vi "RP Read Subset VISA.vi"(6 "Bytes per sample":i32, 7 "Samples per trigger increment":i32=2, 8 "Error In":errorcluster, 9 "Post-trigger samples":u64=11534336 format="0x%x (%d)", 10 "Pre-trigger samples":i32=-100000 format="0x%x (%d)", 11 "VISA resource":refnum<visa-resource-name>) -> (0 "Error Out":errorcluster, 1 "Record start pos":u32=1, 2 "Data stream":string, 3 "VISA resource out":refnum<visa-resource-name>)   [LabVIEW 2024]
uses:
  RP Command.ctl
  RP Status Offsets.ctl
  RP Read Status VISA.vi
  RP Write Command VISA.vi
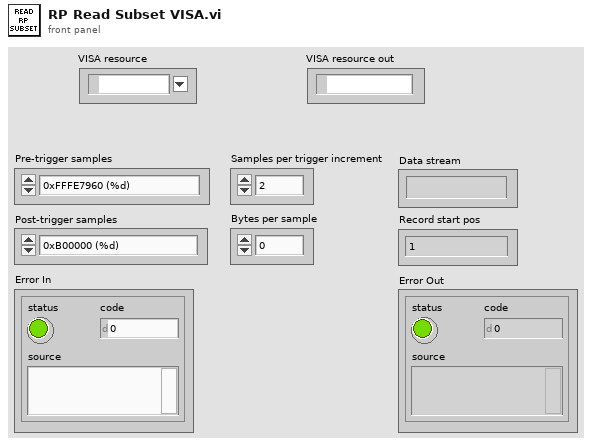
[diagram p1: front panel]
types:
  T1 = typedef "RP Status Offsets.ctl" = u16
  T2 = typedef "RP Command.ctl" = enum16{"Reset", "Read IDN", "Stop server", "Get status", "Get temperature", "Connect client", "Arm", "Software trigger", "Get whole buffer", "Get chunk", "System call", "Get config", "Set config", "Recieve data", "Recieve Calibartion", "Transmit data"}
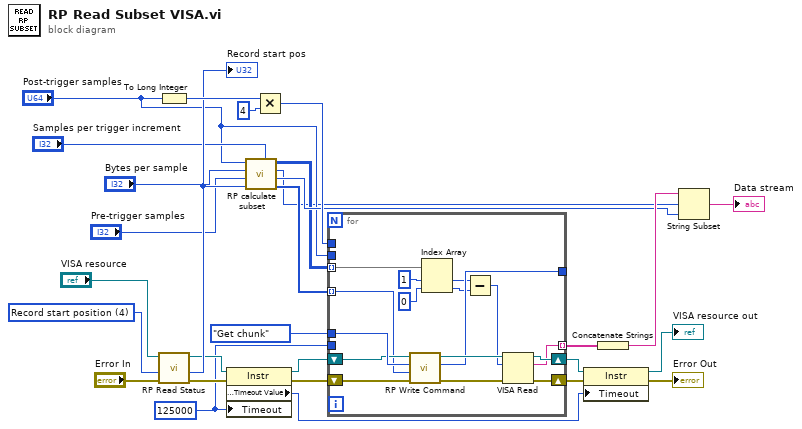
[diagram p0: block diagram]
diagram:
  w25 = T1 4 items=["Writer address"=0, "Record start position"=4, "Trig state etc."=8, "RxFIFO counter"=24, "TxFIFO counter"=28] ("Status offset")
  w2 = u32 125000 ("timeout ms (25000)")
  n1 = To Long Integer(number="Post-trigger samples") -> (32bit integer=w26:i32)
  n2 = call-poly "RP Read Status.vi"("Error In"="Error In", "Status offset"=w25, "VISA resource"="VISA resource") -> ("Error Out"=w9:errorcluster, "Status response"=w24:u32, "VISA resource out"=w11:refnum<visa-resource-name>)  [unwired: 6 in]
  "Record start pos" <- w24
  n3 = property class="Instr"(reference=w11, error in=w9, "Timeout"=w2) -> (reference out=w10:refnum<visa-resource-name>, error out=w8:errorcluster, "General Settings:Timeout Value"=w7:u32)
  n4 = call "RP calculate subset.vi"("Samples per trigger increment"="Samples per trigger increment", "Trigger start position"=w24, "Pre-trigger samples"="Pre-trigger samples", "Bytes per sample"="Bytes per sample", "Post-trigger samples"="Post-trigger samples") -> ("Merged subsets"=w23:u64[], "record length"=w20:i32, "pre-trigger trim"=w1:i32, "Subsets"=w17:i32[][])  [unwired: 3 in]
  n5 = Multiply(x=w26, y=4) -> (x*y=w28:i32)
  n6 = for {
    tunnel: w28 -> [_]
    tunnel: RP_Command."Get chunk" ("Command number") -> [w45]
    tunnel: [w42] -> _
    tunnel: w2 -> [_]
    tunnel: "Post-trigger samples" -> [_]
    shift-right: [w40] -> w4
    shift-left: w8 -> [w39]
    shift-right: [w41] -> w6
    shift-left: w10 -> [w38]
    tunnel: w23 -> [w37] mode=indexing
    tunnel: [w36] -> w22 mode=indexing
    tunnel: w17 -> [w34] mode=indexing
    n7 = call-poly "RP Write Command.vi"("Error In"=w39, "Command payload"=w37, "Command number"=w45, "VISA resource"=w38) -> ("Error Out"=w43:errorcluster, "bytes written"=w42:i32, "VISA resource out"=w44:refnum<visa-resource-name>)  [unwired: 5 in]
    n8 = Index Array(array=w34, index #1=1 ("index"), index #2=0 ("index")) -> (element #1=w33:i32, element #2=w32:i32)
    n9 = Subtract(x=w33, y=w32) -> (x-y=w31:i32)
    n10 = VISA Read(VISA resource name=w44, byte count=w31, error in (no error)=w43) -> (VISA resource name out=w41:refnum<visa-resource-name>, read buffer=w36:string, error out=w40:errorcluster)  [unwired: 1 out]
  }
  n11 = property class="Instr"(reference=w6, error in=w4, "Timeout"=w7) -> (reference out=→"VISA resource out":refnum<visa-resource-name>, error out=→"Error Out":errorcluster)
  n12 = Concatenate Strings(w22) -> (w21:string)
  n13 = String Subset(string=w21, offset (0)=w1, length (rest)=w20) -> (substring=→"Data stream":string)
